vi "99%BWforEXA_Main.vi"() -> ()   [LabVIEW 2016]
panel:
  in  "File name":string
  in  "Path":path
  in  "Catch Screen Shot":bool=TRUE
  in  "Time to wait for trace stablizing (s)":dbl
  in  "Start Test":bool
  in  "Centre Frequency":dbl
  out "Equipment ID":string
  in  "Mode Preset":bool
  in  "VBW Unit":u16(ring) items=["Hz", "KHz", "MHz"]
  in  "RBW Unit":u16(ring) items=["Hz", "KHz", "MHz"]
  in  "Trace Operation":u16(ring) items=["Clear Write", "Average", "Max Hold", "Min Hold"]
  in  "Enable Auto Detector (T: Enable)":bool=TRUE
  in  "Manual Detector Type (0: Average)":i32(ring) items=["Average", "Peak", "Sample", "Negative Peak"]
  in  "Enable Continuous Sweep Mode (F: Disable)":bool
  in  "CENTRE F Unit":u16(ring) items=["Hz", "KHz", "MHz", "GHz"]
  in  "SPAN Unit":u16(ring) items=["Hz", "KHz", "MHz", "GHz"]
  in  "XdB (-26dB)":dbl format="%#_13g"
  in  "Span":dbl=99.0 format="%#.6g"
  in  "Manual Resolution BandWidth":dbl=50880.0
  in  "Enable Auto Sweep Time (T: Enable)":bool=TRUE
  in  "Manual Sweep Time (ms)":dbl=0.265
  in  "Enable Auto Resolution BandWidth (T: Enable)":bool=TRUE
  in  "Enable Auto Video BandWidth (T: Enable)":bool=TRUE
  in  "Manual Video BandWidth":dbl=-14656.0
  in  "Reference Level (0)":dbl
  in  "Amplitude Units (0: dBm)":u16(ring) items=["dBm", "dBmV", "dBmA", "dBuV", "dBuVm", "dBuA", "dBuAm", "dBpt", "dBg", "Volts", "Watts", "Amps"]
  in  "Manual Attenuation (30 dB)":dbl=30.0
  in  "Enable Auto Attenuation (T: Enable)":bool=TRUE
  in  "Reference Level Offset (0 dB)":dbl
  in  "Stop":bool
  in  "Occupied Bandwidth Percent Power (99%)":dbl=99.0 format="%#.6g"
  in  "VISA resource name":refnum<visa-resource-name>
  # "Frequency"
  # "Bandwidth"
  # "Amplitude"
  # "Sweep"
  # "Detector"
  # "Measurement operation"
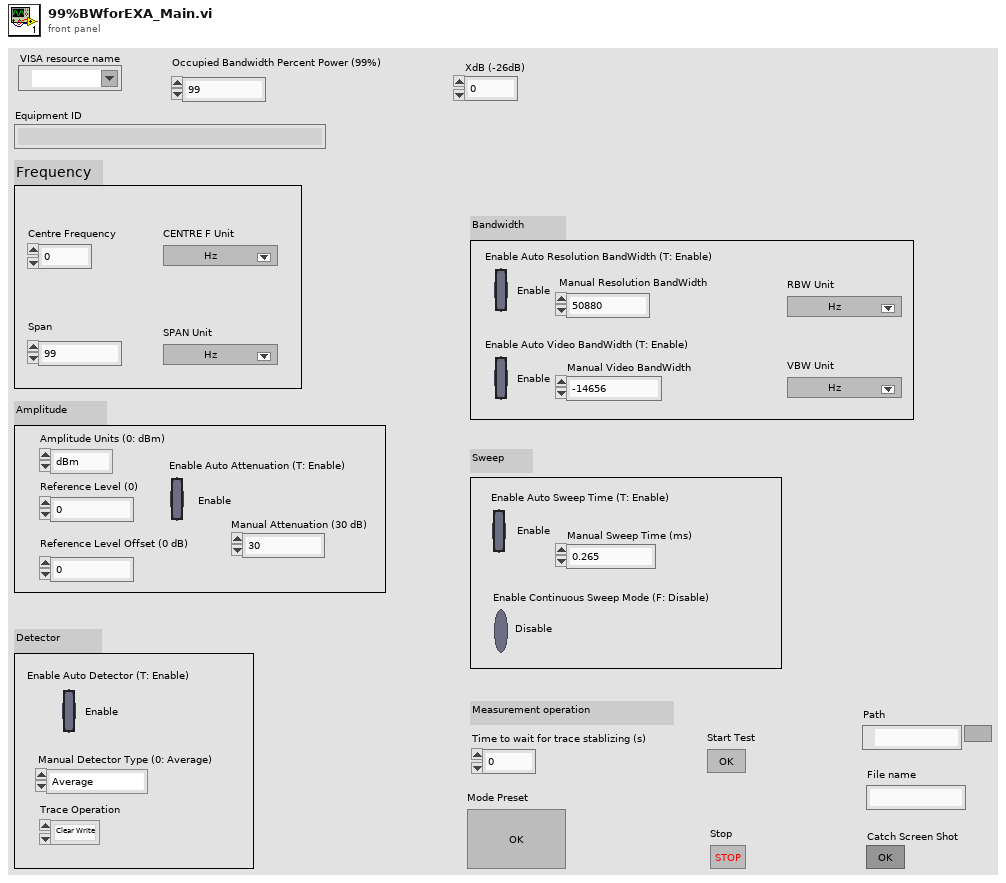
[diagram p1: front panel]
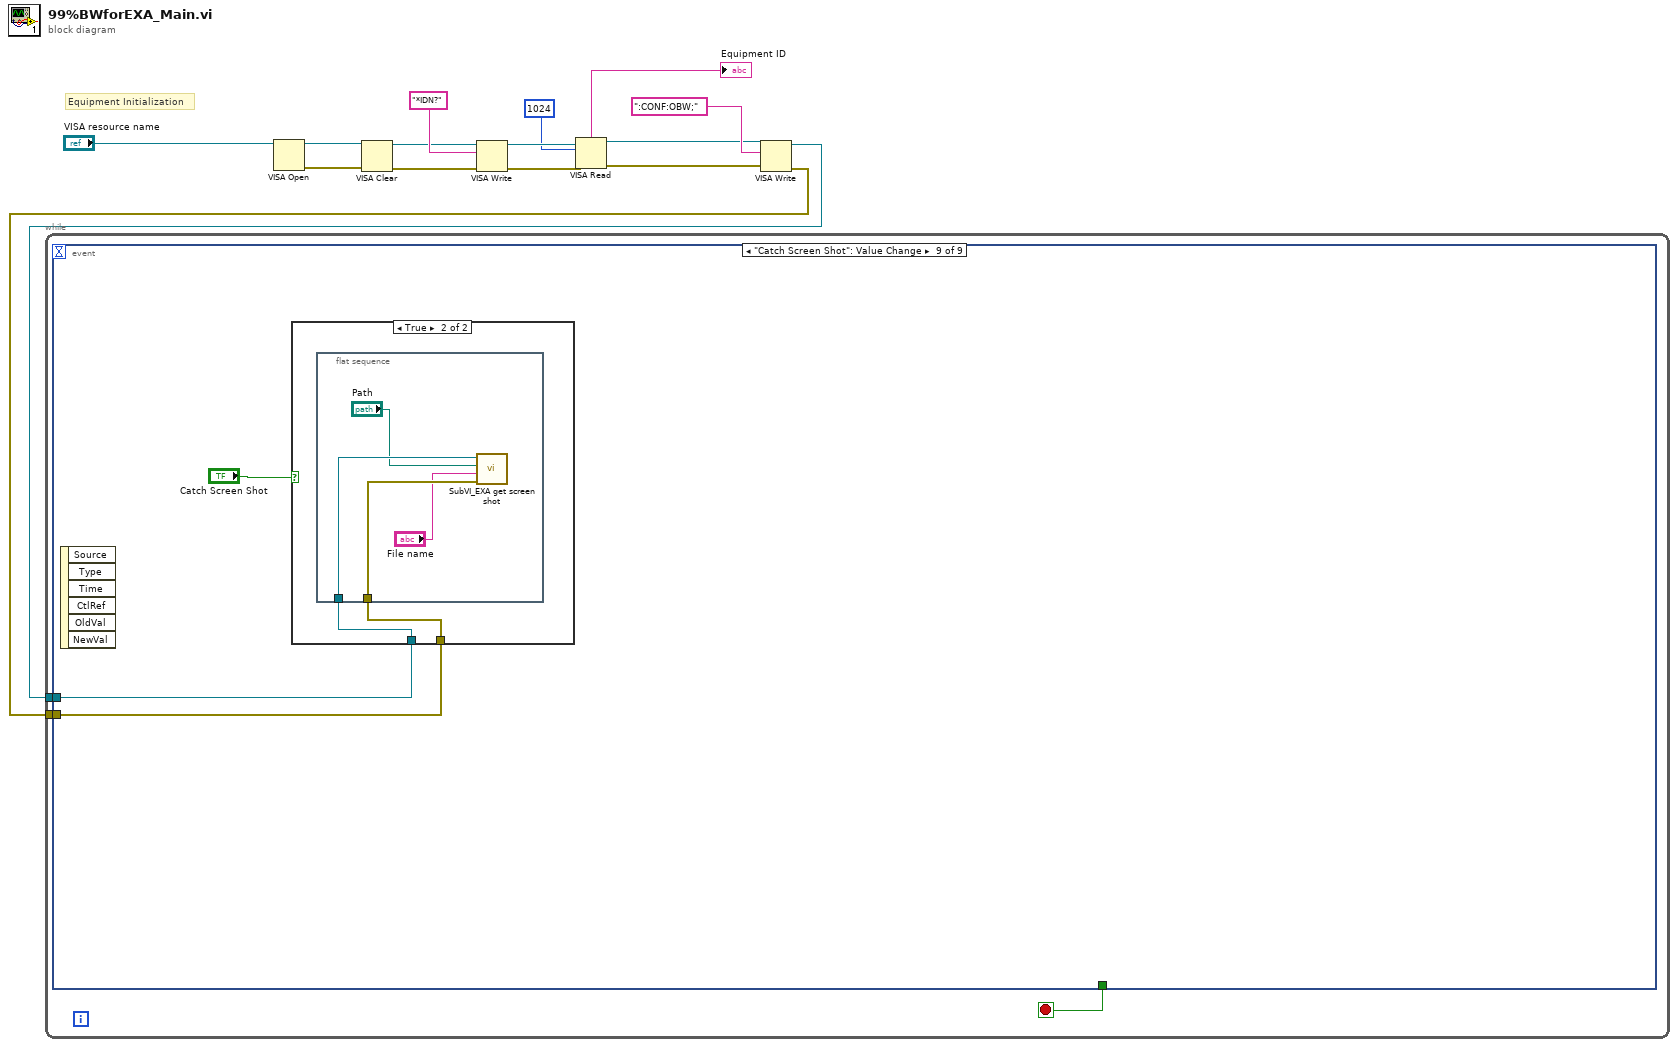
[diagram p0: block diagram]
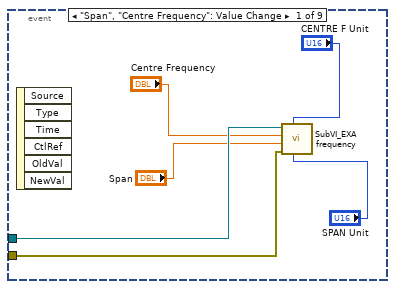
[diagram p2: hidden frame]
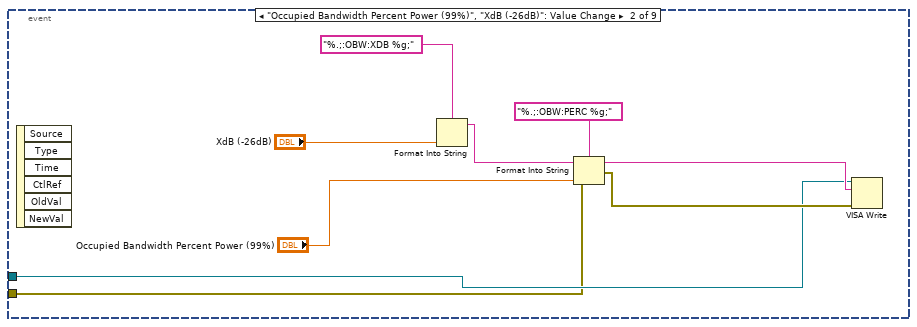
[diagram p3: hidden frame]
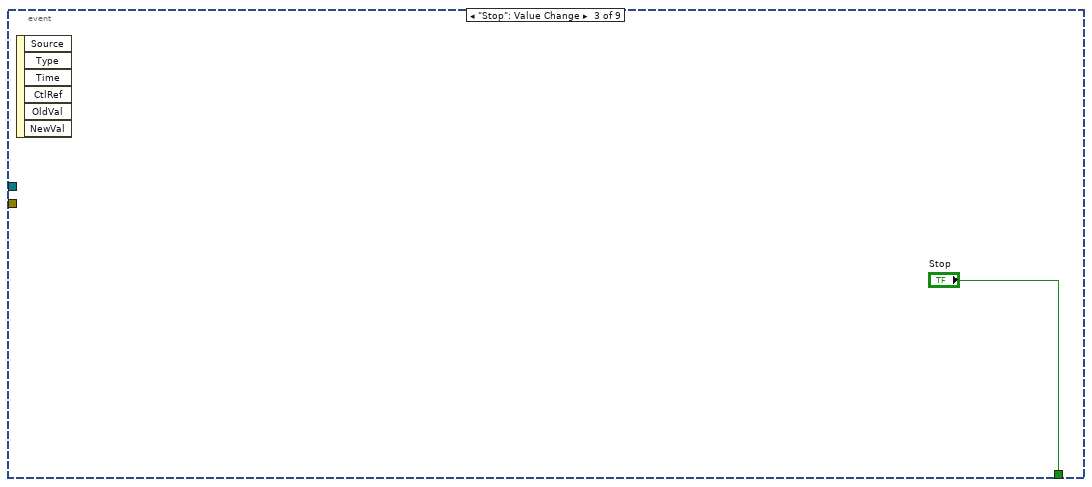
[diagram p4: hidden frame]
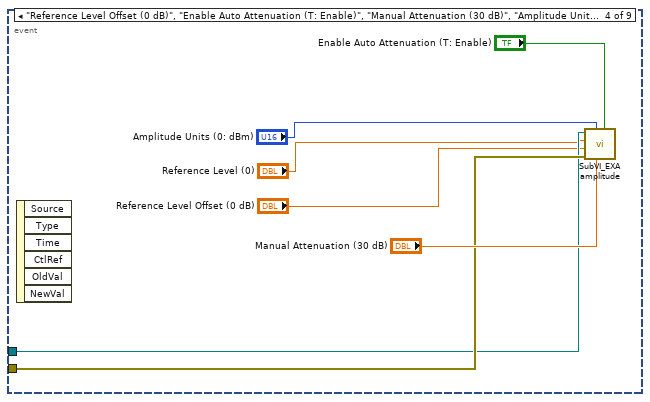
[diagram p5: hidden frame]
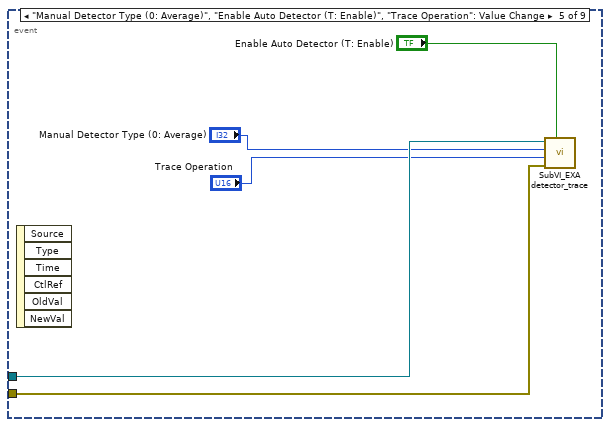
[diagram p6: hidden frame]
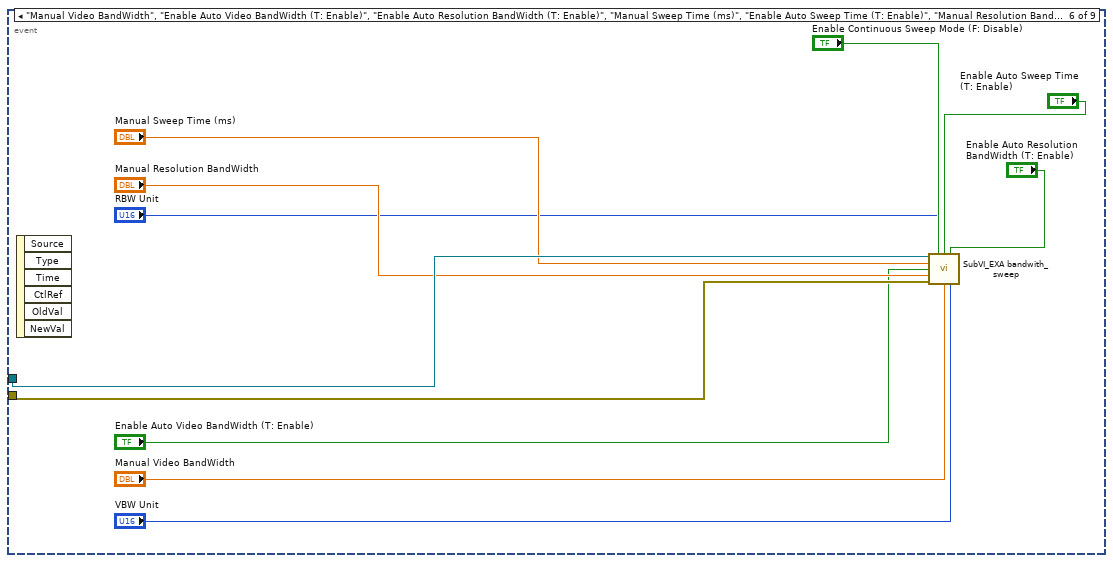
[diagram p7: hidden frame]
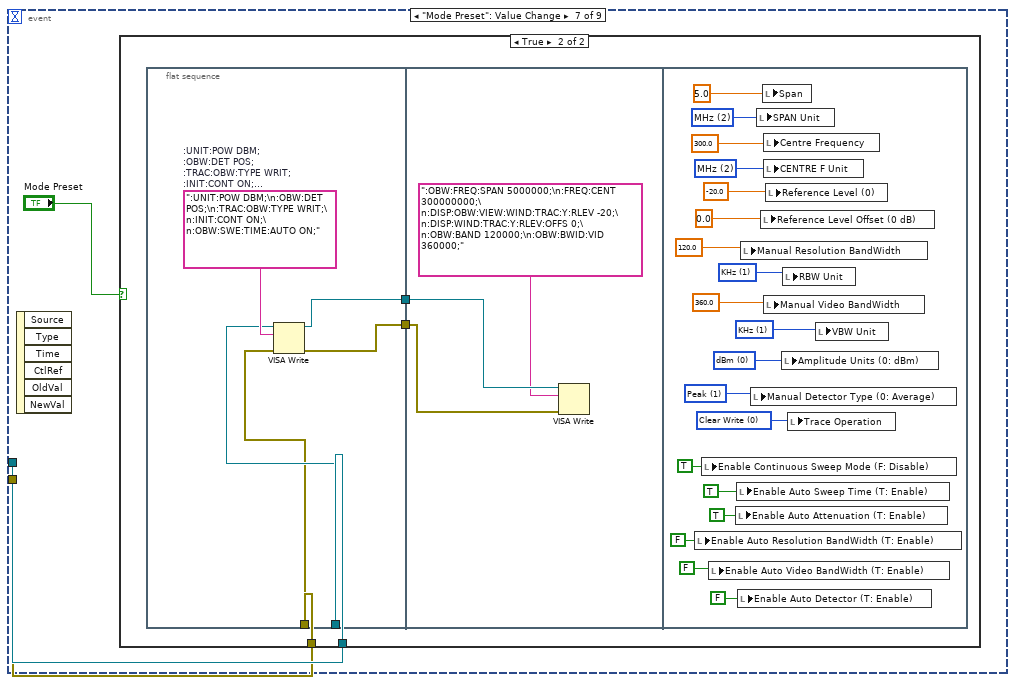
[diagram p8: hidden frame]
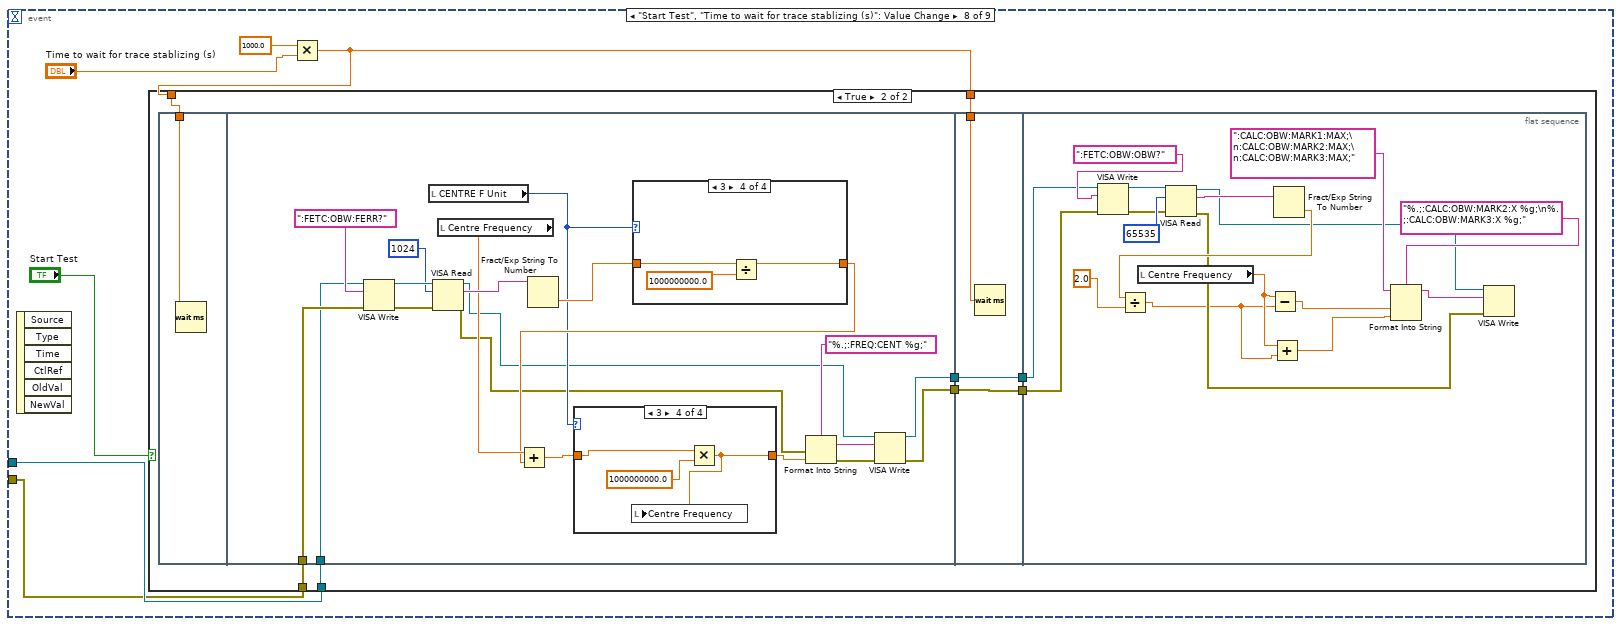
[diagram p10: hidden frame]
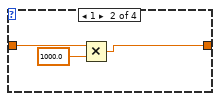
[diagram p13: hidden frame]
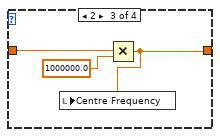
[diagram p14: hidden frame]
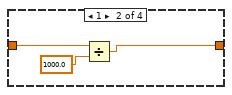
[diagram p16: hidden frame]
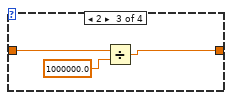
[diagram p17: hidden frame]
diagram:
  # "Equipment Initialization"
  n1 = VISA Open(VISA resource name="VISA resource name") -> (VISA resource name=w12:refnum<visa-resource-name>, error out=w10:errorcluster)  [unwired: 4 in]
  n2 = VISA Clear(VISA resource name=w12, error in (no error)=w10) -> (VISA resource name out=w11:refnum<visa-resource-name>, error out=w9:errorcluster)
  n3 = VISA Write(VISA resource name=w11, write buffer="*IDN?", error in (no error)=w9) -> (VISA resource name out=w6:refnum<visa-resource-name>, error out=w3:errorcluster)  [unwired: 1 out]
  n4 = VISA Read(VISA resource name=w6, byte count=u32 1024, error in (no error)=w3) -> (VISA resource name out=w2:refnum<visa-resource-name>, read buffer=→"Equipment ID":string, error out=w1:errorcluster)  [unwired: 1 out]
  n5 = VISA Write(VISA resource name=w2, write buffer=":CONF:OBW;" ("initial string"), error in (no error)=w1) -> (VISA resource name out=w8:refnum<visa-resource-name>, error out=w7:errorcluster)  [unwired: 1 out]
  n6 = while {
    tunnel: w8 -> [w18]
    tunnel: w7 -> [w17]
    stop <- w16 stop-if-true
    n7 = event shown="[8] \"Catch Screen Shot\": Value Change" {
      selector: _ -> [_ _ _ _ _ _ _ _ _]
      dyn-events: _ -> [_ _ _ _ _ _ _ _ _]
      timeout: _ -> [_ _ _ _ _ _ _ _ _]
      tunnel: w18 -> [w23 w29 _ w37 w44 w54 w59 w96 w170]
      tunnel: w17 -> [w22 w28 _ w38 w45 w55 w58 w95 w169]
      tunnel: [_ _ "Stop" _ _ _ _ _ _] -> w16
      event "Span", "Centre Frequency": Value Change {
        n8 = event-data() -> ()  [unwired: 1 in, 6 out]
        n9 = call "SubVI_EXA frequency.vi"("SPAN Unit"="SPAN Unit", "CENTRE F Unit"="CENTRE F Unit", "error in (no error)"=w22, "Span"="Span", "Centre Frequency"="Centre Frequency", "VISA Refnum in"=w23) -> ()  [unwired: 4 in, 2 out]
      }
      event "Occupied Bandwidth Percent Power (99%)", "XdB (-26dB)": Value Change {
        n10 = event-data() -> ()  [unwired: 1 in, 6 out]
        n11 = Format Into String(format string="%.;:OBW:XDB %g;", "XdB (-26dB)") -> (resulting string=w25:string)  [unwired: 2 in, 1 out]
        n12 = Format Into String(format string="%.;:OBW:PERC %g;", initial string=w25, error in=w28, "Occupied Bandwidth Percent Power (99%)") -> (resulting string=w33:string, error out=w32:errorcluster)
        n13 = VISA Write(VISA resource name=w29, write buffer=w33, error in (no error)=w32) -> ()  [unwired: 3 out]
      }
      event "Stop": Value Change {
        n14 = event-data() -> ()  [unwired: 1 in, 6 out]
      }
      event "Reference Level Offset (0 dB)", "Enable Auto Attenuation (T: Enable)", "Manual Attenuation (30 dB)", "Amplitude Units (0: dBm)", "Reference Level (0)": Value Change {
        n15 = event-data() -> ()  [unwired: 1 in, 6 out]
        n16 = call "SubVI_EXA amplitude.vi"("Enable Auto Attenuation (T: Enable)"="Enable Auto Attenuation (T: Enable)", "Manual Attenuation (30 dB)"="Manual Attenuation (30 dB)", "Amplitude Units (0: dBm)"="Amplitude Units (0: dBm)", "error in (no error)"=w38, "Reference Level Offset (0 dB)"="Reference Level Offset (0 dB)", "Reference Level (0)"="Reference Level (0)", "VISA Refnum in"=w37) -> ()  [unwired: 3 in, 2 out]
      }
      event "Manual Detector Type (0: Average)", "Enable Auto Detector (T: Enable)", "Trace Operation": Value Change {
        n17 = event-data() -> ()  [unwired: 1 in, 6 out]
        n18 = call "SubVI_EXA detector_trace.vi"("Enable Auto Detector (T: Enable)"="Enable Auto Detector (T: Enable)", "error in (no error)"=w45, "Trace Operation"="Trace Operation", "Detector"="Manual Detector Type (0: Average)", "VISA Refnum in"=w44) -> ()  [unwired: 5 in, 2 out]
      }
      event "Manual Video BandWidth", "Enable Auto Video BandWidth (T: Enable)", "Enable Auto Resolution BandWidth (T: Enable)", "Manual Sweep Time (ms)", "Enable Auto Sweep Time (T: Enable)", "Manual Resolution BandWidth", "Enable Continuous Sweep Mode (F: Disable)": Value Change {
        n19 = event-data() -> ()  [unwired: 1 in, 6 out]
        n20 = call "SubVI_EXA bandwith_sweep.vi"("VISA Refnum in"=w54, "Enable Continuous Sweep Mode (F: Disable)"="Enable Continuous Sweep Mode (F: Disable)", "Enable Auto Sweep Time (T: Enable)"="Enable Auto Sweep Time (T: Enable)", "Enable Auto Resolution BandWidth (T: Enable)"="Enable Auto Resolution BandWidth (T: Enable)", "Manual Sweep Time (265 ms)"="Manual Sweep Time (ms)", "Enable Auto Video BandWidth (T: Enable)"="Enable Auto Video BandWidth (T: Enable)", "Manual Resolution BandWidth (3 MHz)"="Manual Resolution BandWidth", "error in (no error)"=w55, "RBW Unit"="RBW Unit", "Manual Video BandWidth (3 MHz)"="Manual Video BandWidth", "VBW Unit"="VBW Unit") -> ()  [unwired: 3 in, 2 out]
      }
      event "Mode Preset": Value Change {
        n21 = event-data() -> ()  [unwired: 1 in, 6 out]
        n22 = case shown="True" "Mode Preset" {
          tunnel: w59 -> [_ w64]
          tunnel: w58 -> [_ w63]
          frame False {
          }
          frame True {
            n23 = flat-sequence {
              tunnel: w64 -> [w68]
              tunnel: w63 -> [w67]
              tunnel: [w66] -> w62
              tunnel: [w65] -> w61
              tunnel: w62 -> [w72]
              tunnel: w61 -> [w71]
              frame #0 {
                w69 = ":UNIT:POW DBM;\n:OBW:DET POS;\n:TRAC:OBW:TYPE WRIT;\n:INIT:CONT ON;\n:OBW:SWE:TIME:AUTO ON;"  # :UNIT:POW DBM; :OBW:DET POS; :TRAC:OBW:TYPE WRIT; :INIT:CONT ON; :OBW:SWE:TIME:AUTO ON;
                n24 = VISA Write(VISA resource name=w68, write buffer=w69, error in (no error)=w67) -> (VISA resource name out=w66:refnum<visa-resource-name>, error out=w65:errorcluster)  [unwired: 1 out]
              }
              frame #1 {
                n25 = VISA Write(VISA resource name=w72, write buffer=":OBW:FREQ:SPAN 5000000;\n:FREQ:CENT 300000000;\n:DISP:OBW:VIEW:WIND:TRAC:Y:RLEV -20;\n:DISP:WIND:TRAC:Y:RLEV:OFFS 0;\n:OBW:BAND 120000;\n:OBW:BWID:VID 360000;", error in (no error)=w71) -> ()  [unwired: 3 out]
              }
              frame #2 {
                w80 = u16 0 items=["Clear Write", "Average", "Max Hold", "Min Hold"] ("Trace Operation")
                w81 = 1 items=["Average", "Peak", "Sample", "Negative peak"] ("Manual Detector Type (0: Average)")
                w82 = u16 0 items=["dBm", "dBmV", "dBmA", "dBuV", "dBuVm", "dBuA", "dBuAm", "dBpt", "dBg", "Volts", "Watts", "Amps"] ("Amplitude Units (0: dBm)")
                w83 = u16 1 items=["Hz", "KHz", "MHz"] ("VBW Unit")
                w85 = u16 1 items=["Hz", "KHz", "MHz"] ("RBW Unit")
                w89 = u16 2 items=["Hz", "KHz", "MHz", "GHz"] ("CENTRE F Unit")
                w90 = u16 2 items=["Hz", "KHz", "MHz", "GHz"] ("SPAN Unit")
                n26 = local write "Enable Auto Resolution BandWidth (T: Enable)"(FALSE ("Enable Auto Resolution BandWidth (T: Enable)")) -> ()
                n27 = local write "Enable Continuous Sweep Mode (F: Disable)"(TRUE ("Enable Continuous Sweep Mode (F: Disable)")) -> ()
                n28 = local write "Enable Auto Video BandWidth (T: Enable)"(FALSE ("Enable Auto Video BandWidth (T: Enable)")) -> ()
                n29 = local write "Enable Auto Attenuation (T: Enable)"(TRUE ("Enable Auto Attenuation (T: Enable)")) -> ()
                n30 = local write "Enable Auto Sweep Time (T: Enable)"(TRUE ("Enable Auto Sweep Time (T: Enable)")) -> ()
                n31 = local write "Enable Auto Detector (T: Enable)"(FALSE ("Enable Auto Detector (T: Enable)")) -> ()
                n32 = local write "Manual Resolution BandWidth"(120.0 ("Manual Resolution BandWidth (3 MHz)")) -> ()
                n33 = local write "Manual Detector Type (0: Average)"(w81) -> ()
                n34 = local write "SPAN Unit"(w90) -> ()
                n35 = local write "Reference Level Offset (0 dB)"(0.0 ("Reference Level Offset (0 dB)")) -> ()
                n36 = local write "Span"(5.0 ("Span")) -> ()
                n37 = local write "Centre Frequency"(300.0 ("Centre Frequency")) -> ()
                n38 = local write "CENTRE F Unit"(w89) -> ()
                n39 = local write "Manual Video BandWidth"(360.0 ("Manual Video BandWidth (3 MHz)")) -> ()
                n40 = local write "Reference Level (0)"(-20.0 ("Reference Level (0)")) -> ()
                n41 = local write "Amplitude Units (0: dBm)"(w82) -> ()
                n42 = local write "RBW Unit"(w85) -> ()
                n43 = local write "Trace Operation"(w80) -> ()
                n44 = local write "VBW Unit"(w83) -> ()
              }
            }
          }
        }
      }
      event "Start Test", "Time to wait for trace stablizing (s)": Value Change {
        n45 = event-data() -> ()  [unwired: 1 in, 6 out]
        n46 = Multiply(x=1000.0, y="Time to wait for trace stablizing (s)") -> (x*y=w92:dbl)
        n47 = case shown="True" "Start Test" {
          tunnel: w96 -> [_ w104]
          tunnel: w95 -> [_ w105]
          tunnel: w92 -> [_ w99]
          tunnel: w92 -> [_ w98]
          frame False {
          }
          frame True {
            n48 = flat-sequence {
              tunnel: w99 -> [w106]
              tunnel: w105 -> [w108]
              tunnel: w104 -> [w107]
              tunnel: [w110] -> w103
              tunnel: [w109] -> w101
              tunnel: w103 -> [w149]
              tunnel: [w149] -> w102
              tunnel: w101 -> [w148]
              tunnel: [w148] -> w100
              tunnel: w98 -> [w147]
              tunnel: w102 -> [w160]
              tunnel: w100 -> [w159]
              frame #0 {
                n49 = Wait (ms)(milliseconds to wait=w106) -> ()  [unwired: 1 out]
              }
              frame #1 {
                n50 = VISA Write(VISA resource name=w107, write buffer=":FETC:OBW:FERR?", error in (no error)=w108) -> (VISA resource name out=w125:refnum<visa-resource-name>, error out=w124:errorcluster)  [unwired: 1 out]
                n51 = local read "CENTRE F Unit"() -> (w117:u16)
                n52 = VISA Read(VISA resource name=w125, byte count=u32 1024, error in (no error)=w124) -> (VISA resource name out=w113:refnum<visa-resource-name>, read buffer=w122:string, error out=w112:errorcluster)  [unwired: 1 out]
                n53 = local read "Centre Frequency"() -> (w120:dbl)
                n54 = Fract/Exp String To Number(string=w122) -> (number=w121:dbl)  [unwired: 3 in, 1 out]
                n55 = case shown="3" w117 {
                  tunnel: w121 -> [w137 w140 w143 w146]
                  tunnel: [w137 w139 w142 w145] -> w119
                  frame 0, Default {
                  }
                  frame 1 {
                    n56 = Divide(x=w140, y=1000.0) -> (x/y=w139:dbl)
                  }
                  frame 2 {
                    n57 = Divide(x=w143, y=1000000.0) -> (x/y=w142:dbl)
                  }
                  frame 3 {
                    n58 = Divide(x=w146, y=1000000000.0) -> (x/y=w145:dbl)
                  }
                }
                n59 = Add(x=w120, y=w119) -> (x+y=w116:dbl)
                n60 = case shown="3" w117 {
                  tunnel: w116 -> [w127 w130 w133 w136]
                  tunnel: [w127 w128 w131 w134] -> w115
                  frame 0, Default {
                  }
                  frame 1 {
                    n61 = Multiply(x=w130, y=1000.0) -> (x*y=w128:dbl)
                  }
                  frame 2 {
                    n62 = Multiply(x=w133, y=1000000.0) -> (x*y=w131:dbl)
                    n63 = local write "Centre Frequency"(w131) -> ()
                  }
                  frame 3 {
                    n64 = Multiply(x=w136, y=1000000000.0) -> (x*y=w134:dbl)
                    n65 = local write "Centre Frequency"(w134) -> ()
                  }
                }
                n66 = Format Into String(format string="%.;:FREQ:CENT %g;", error in=w112, w115) -> (resulting string=w111:string, error out=w114:errorcluster)  [unwired: 1 in]
                n67 = VISA Write(VISA resource name=w113, write buffer=w111, error in (no error)=w114) -> (VISA resource name out=w110:refnum<visa-resource-name>, error out=w109:errorcluster)  [unwired: 1 out]
              }
              frame #2 {
                n68 = Wait (ms)(milliseconds to wait=w147) -> ()  [unwired: 1 out]
              }
              frame #3 {
                n69 = VISA Write(VISA resource name=w160, write buffer=":FETC:OBW:OBW?", error in (no error)=w159) -> (VISA resource name out=w162:refnum<visa-resource-name>, error out=w161:errorcluster)  [unwired: 1 out]
                n70 = local read "Centre Frequency"() -> (w152:dbl)
                n71 = VISA Read(VISA resource name=w162, byte count=u32 65535, error in (no error)=w161) -> (VISA resource name out=w154:refnum<visa-resource-name>, read buffer=w165:string, error out=w153:errorcluster)  [unwired: 1 out]
                n72 = Fract/Exp String To Number(string=w165) -> (number=w163:dbl)  [unwired: 3 in, 1 out]
                n73 = Divide(x=w163, y=2.0) -> (x/y=w151:dbl)
                n74 = Subtract(x=w152, y=w151) -> (x-y=w158:dbl)
                n75 = Add(x=w152, y=w151) -> (x+y=w150:dbl)
                n76 = Format Into String(format string="%.;:CALC:OBW:MARK2:X %g;\n%.;:CALC:OBW:MARK3:X %g;", initial string=":CALC:OBW:MARK1:MAX;\n:CALC:OBW:MARK2:MAX;\n:CALC:OBW:MARK3:MAX;", w158, w150) -> (resulting string=w155:string)  [unwired: 1 in, 1 out]
                n77 = VISA Write(VISA resource name=w154, write buffer=w155, error in (no error)=w153) -> ()  [unwired: 3 out]
              }
            }
          }
        }
      }
      event "Catch Screen Shot": Value Change {
        n78 = event-data() -> ()  [unwired: 1 in, 6 out]
        n79 = case shown="True" "Catch Screen Shot" {
          tunnel: w170 -> [_ w172]
          tunnel: w169 -> [_ w171]
          frame False {
          }
          frame True {
            n80 = flat-sequence {
              tunnel: w172 -> [w176]
              tunnel: w171 -> [w175]
              frame #0 {
                n81 = call "SubVI_EXA get screen shot.vi"("error in (no error)"=w175, "File name"="File name", "Path"="Path", "VISA resource in"=w176) -> ()  [unwired: 6 in, 2 out]
              }
            }
          }
        }
      }
    }
  }
